vi "Show Child In Sub Panel.vi"(8 "error in (no error)":errorcluster, 10 "Child name":string, 11 "ActorMeter in":refnum<class "ActorMeter.lvclass">) -> (0 "error out":errorcluster, 3 "ActorMeter out":refnum<class "ActorMeter.lvclass">)   [LabVIEW 2014, in "ActorMeter.lvclass"]
uses:
  ActorMeter.lvclass
  ActorMeter.lvclass/ActorMeter.ctl
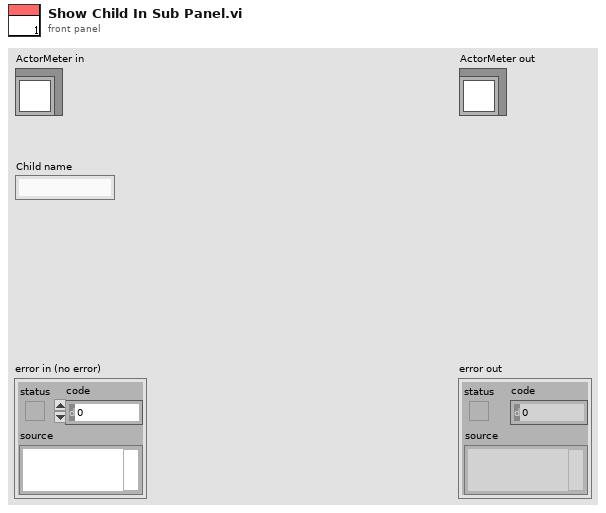
[diagram p1: front panel]
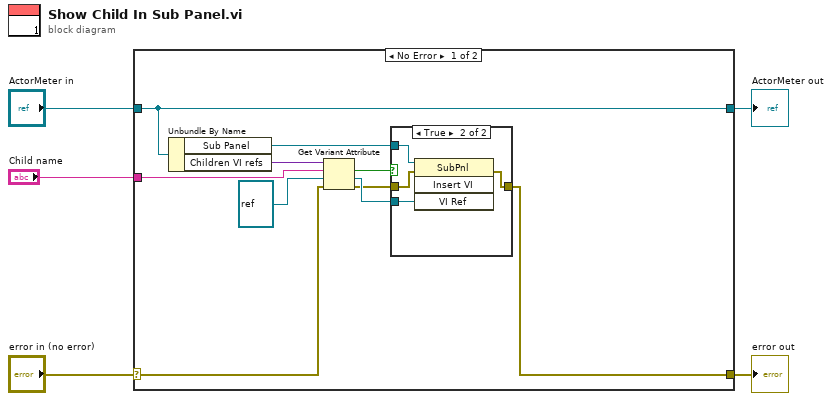
[diagram p0: block diagram]
diagram:
  n1 = case shown="No Error" "error in (no error)" {
    selector: "error in (no error)" -> [w7 w22]
    tunnel: [w6 w22] -> w4
    tunnel: [w15 w21] -> w2
    tunnel: "ActorMeter in" -> [w15 w21]
    tunnel: "Child name" -> [w8 _]
    frame No Error {
      n2 = Unbundle By Name(w15) -> ("Sub Panel"=w9:refnum<vi>, "Children VI refs"=w14:variant)
      n3 = Get Variant Attribute(Variant=w14, name=w8, default value (empty Variant)=refnum<vi> refnum ("VI ref"), error in=w7) -> (found=w13:bool, value=w11:refnum<vi>, error out=w10:errorcluster)  [unwired: 1 out]
      n4 = case shown="True" w13 {
        tunnel: w11 -> [_ w20]
        tunnel: w10 -> [w16 w19]
        tunnel: [w16 w18] -> w6
        tunnel: w9 -> [_ w17]
        frame False {
        }
        frame True {
          n5 = invoke class="SubPnl" method="Insert VI"(reference=w17, error in=w19, "VI Ref"=w20) -> (error out=w18:errorcluster)  [unwired: 1 in, 3 out]
        }
      }
    }
    frame Error {
    }
  }
  "error out" <- w4
  "ActorMeter out" <- w2
